vi "重构数组.vi"() -> ()   [LabVIEW 2010]
panel:
  out "重构的\n数组":i32[][](array[numeric])
  out "重构的\n数组":i32[](array[numeric])
  out "重构的\n数组":i32[][](array[numeric])
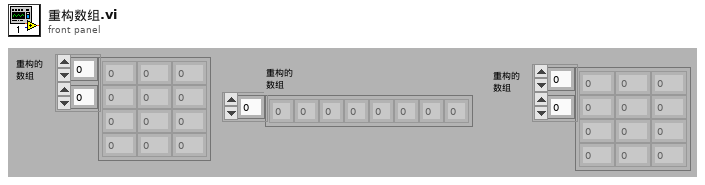
[diagram p1: front panel]
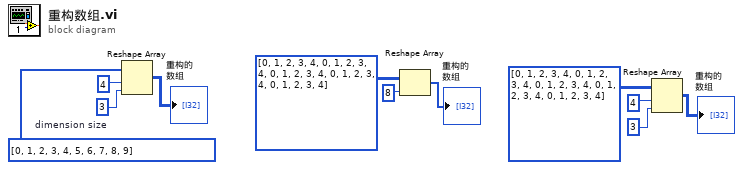
[diagram p0: block diagram]
diagram:
  w9 = 4  # dimension size
  n1 = Reshape Array "Reshape Array"(i32[] [0, 1, 2, 3, 4, 5, 6, 7, 8, 9] ("Array"), w9, 3 ("dimension size")) -> (→"重构的\n数组":i32[][])
  n2 = Reshape Array(i32[][] [[0, 1, 2, 3, 4], [0, 1, 2, 3, 4], [0, 1, 2, 3, 4], [0, 1, 2, 3, 4], [0, 1, 2, 3, 4]] ("Array"), 8 ("dimension size")) -> (→"重构的\n数组":i32[])
  n3 = Reshape Array(i32[][] [[0, 1, 2, 3, 4], [0, 1, 2, 3, 4], [0, 1, 2, 3, 4], [0, 1, 2, 3, 4], [0, 1, 2, 3, 4]] ("Array"), 4 ("dimension size"), 3 ("dimension size")) -> (→"重构的\n数组":i32[][])
